vi "Extract from Table.vi"(9 "Search For":string, 11 "Fun Table":string[][](table)) -> (2 "Filename":string)   [LabVIEW 2009]
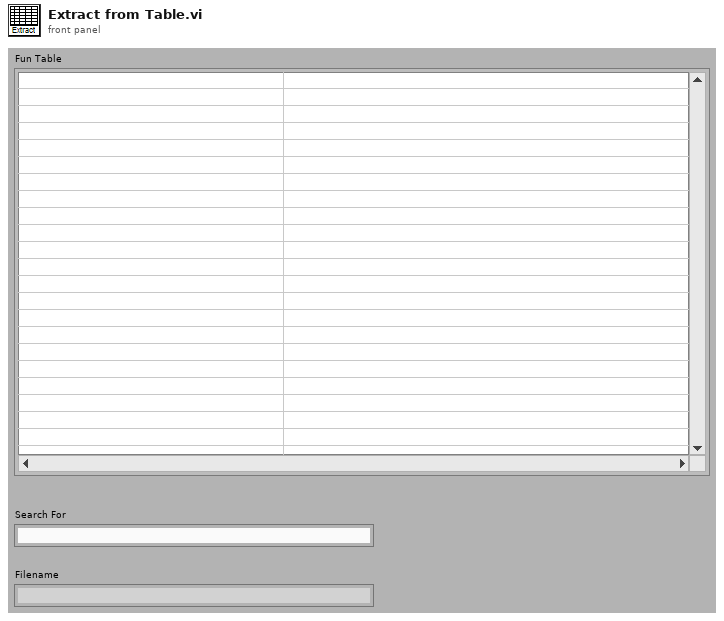
[diagram p1: front panel]
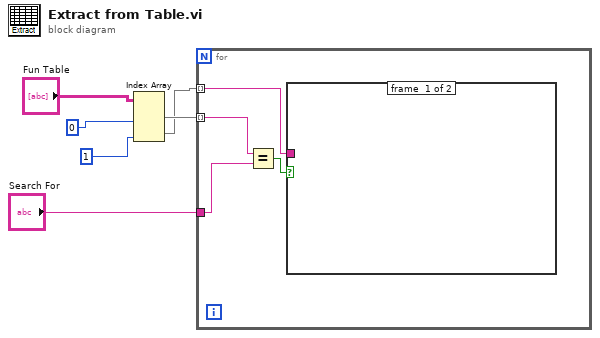
[diagram p0: block diagram]
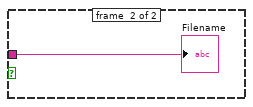
[diagram p2: hidden frame]
diagram:
  n1 = Index Array(array="Fun Table", index (col) #1=0, index (col) #2=1) -> (element #1=w4:string[], element #2=w1:string[])  [unwired: 2 in]
  n2 = for {
    tunnel: w4 -> [w10] mode=indexing
    tunnel: "Search For" -> [w9]
    tunnel: w1 -> [w7] mode=indexing
    n3 = Equal?(x=w10, y=w9) -> (x = y?=w8:bool)
    n4 = case shown="True" w8 {
      tunnel: w7 -> [_ w11]
      frame #0 {
      }
      frame #1 {
        "Filename" <- w11
      }
    }
  }
